vi "Set Parameter Properties.vi"(0 "custom device ref in":T1=18446744073709551615 format="%.0x", 1 "port sessions":T2 {"portConfiguration"."Rx_UDP"."Tx_UDP"."FilterMode" items=["FDX_RX_VL_FLT_DIS", "FDX_RX_VL_FLT_ENA ", "FDX_RX_VL_FLT_ENA_INV"]; "portConfiguration"."Rx_UDP"."Tx_UDP"."VLBufSize" format="%.0x"; "portConfiguration"."Rx_UDP"."Tx_UDP"."VerificationMode" items=["FDX_RX_VL_CHECK_ENA_DEFAULT"=65535, "FDX_RX_VL_CHECK_REDMAM"=16, "DX_RX_VL_CHECK_TRAFIC"=8, "FDX_RX_VL_CHECK_FRAMESIZE"=4, "FDX_RX_VL_CHECK_SNINTEG"=2, "FDX_RX_VL_CHECK_INVPAC"=1, "FDX_RX_VL_CHECK_DISA"=0]; "portConfiguration"."Tx_UDP"."tx_udp_setup"."interfaceID" format="%.0b"; "portConfiguration"."Tx_UDP"."tx_udp_setup"."NetSelect" items=["FDX_TX_FRAME_DLY_A"=0, "FDX_TX_FRAME_DLY_B"=1, "FDX_TX_FRAME_BOTH "=3, "FDX_TX_FRAME_ONLY_A"=4, "FDX_TX_FRAME_ONLY_B "=5]; "portConfiguration"."Rx_Monitor"."Strobe" items=["FDX_MON_STROBE_DIS", "FDX_MON_STROBE_STOP", "FDX_MON_STROBE_START"]; "portConfiguration"."Rx_Monitor"."CaptureMode" items=["FDX_MON_SINGLE ", "FDX_MON_CONTINUOUS", "FDX_MON_SELECTIVE", "FDX_MON_RECORDING", "FDX_MON_REROS", "FDX_MON_HMU"]; "portConfiguration"."Rx_Monitor"."DefaultCronoMode" items=["FDX_RX_DEFAULT_ENA_CNT", "FDX_RX_DEFAULT_MON_ENA_ALL", "FDX_RX_DEFAULT_MON_ENA_GOOD"]; "portConfiguration"."Tx_Generic"."Frame Headers"."Frame header"."PhysErrorInjection" items=["FDX_TX_FRAME_ERR_OFF", "FDX_TX_FRAME_ERR_CRC", "FDX_TX_FRAME_ERR_ALI", "FDX_TX_FRAME_ERR_PRE", "FDX_TX_FRAME_ERR_PHY"]; "portConfiguration"."Tx_Generic"."Frame Headers"."Frame header"."PayloadGenerationMode" items=["FDX_TX_FRAME_PGM_USER", "FDX_TX_FRAME_PGM_IP_PART", "FDX_TX_FRAME_PGM_IP_PART_TT", "FDX_TX_FRAME_PGM_IP_FULL", "FDX_TX_FRAME_PGM_IP_FULL_TT"]; "portConfiguration"."Tx_Generic"."Frame Headers"."Frame header"."PayloadBufferMode" items=["FDX_TX_FRAME_PBM_STD", "FDX_TX_FRAME_PBM_MAC", "FDX_TX_FRAME_PBM_UDP", "FDX_TX_FRAME_PBM_FULL"]; "portConfiguration"."Tx_Generic"."Frame Headers"."Frame header"."NetSelect" items=["FDX_TX_FRAME_DLY_A"=0, "FDX_TX_FRAME_DLY_B"=1, "FDX_TX_FRAME_BOTH "=3, "FDX_TX_FRAME_ONLY_A"=4, "FDX_TX_FRAME_ONLY_B "=5]; "portConfiguration"."Tx_Generic"."Frame Headers"."Frame header"."FrameStartMode" items=["FDX_TX_FRAME_START_IFG", "FDX_TX_FRAME_START_PGWT", "FDX_TX_FRAME_START_TRG", "FDX_TX_FRAME_START_TRG_D"]; "portConfiguration"."Tx_Generic"."tx_generic_setup"."StartMode" items=["FDX_STOP", "FDX_START", "FDX_START_TRG", "FDX_START_TIME"]; "boardSetup"."portConfig" items=["FDX_SINGLE", "FDX_REDUNDANT"]; "boardSetup"."portSpeed" items=["FDX_100MBIT", "FDX_10MBIT", "FDX_AUTO_100MBIT", "FDX_AUTO_10MBIT", "FDX_AUTO_ERROR", "FDX_1000MBIT"]}, 3 "error in":errorcluster) -> (7 "custom device ref out":T1=18446744073709551615 format="%.0x", 10 "error out":errorcluster)   [LabVIEW 2020, in "AIM ARINC 664 Scripting.lvlib"]
uses:
  AIM ARINC 664 Scripting.lvlib
  Import/_typedefs/Board Top Level Configuration.ctl
  Import/_typedefs/board_setup.ctl
  Import/_typedefs/port_configuration.ctl
  Import/_typedefs/port_setup.ctl
  Import/_typedefs/session_tx_generic.ctl
  Import/_typedefs/tx_generic_setup.ctl
  Import/_typedefs/frame_tx_generic.ctl
  Import/_typedefs/frame_tx_generic_seqNumberInit.ctl
  Import/_typedefs/frame_tx_generic_seqNumberOffset.ctl
  Import/_typedefs/frame_parameter.ctl
  Import/_typedefs/frame_parameter_definition.ctl
  Shared/Encoding (Arinc664).ctl
  Import/_typedefs/port_tx_udp_comm.ctl
  Import/_typedefs/port_tx_udp_sap.ctl
  Import/_typedefs/rx_udp_setup.ctl
  Import/_typedefs/port_rx_udp_comm.ctl
  Import/_typedefs/port_rx_udp_sap.ctl
  <vilib>/NI VeriStand/Custom Device API/Custom Device Item Ref.ctl
  Import/AIM ARINC 664 Import.lvlib
  <vilib>/NI VeriStand/Custom Device API/Custom Device API.lvlib
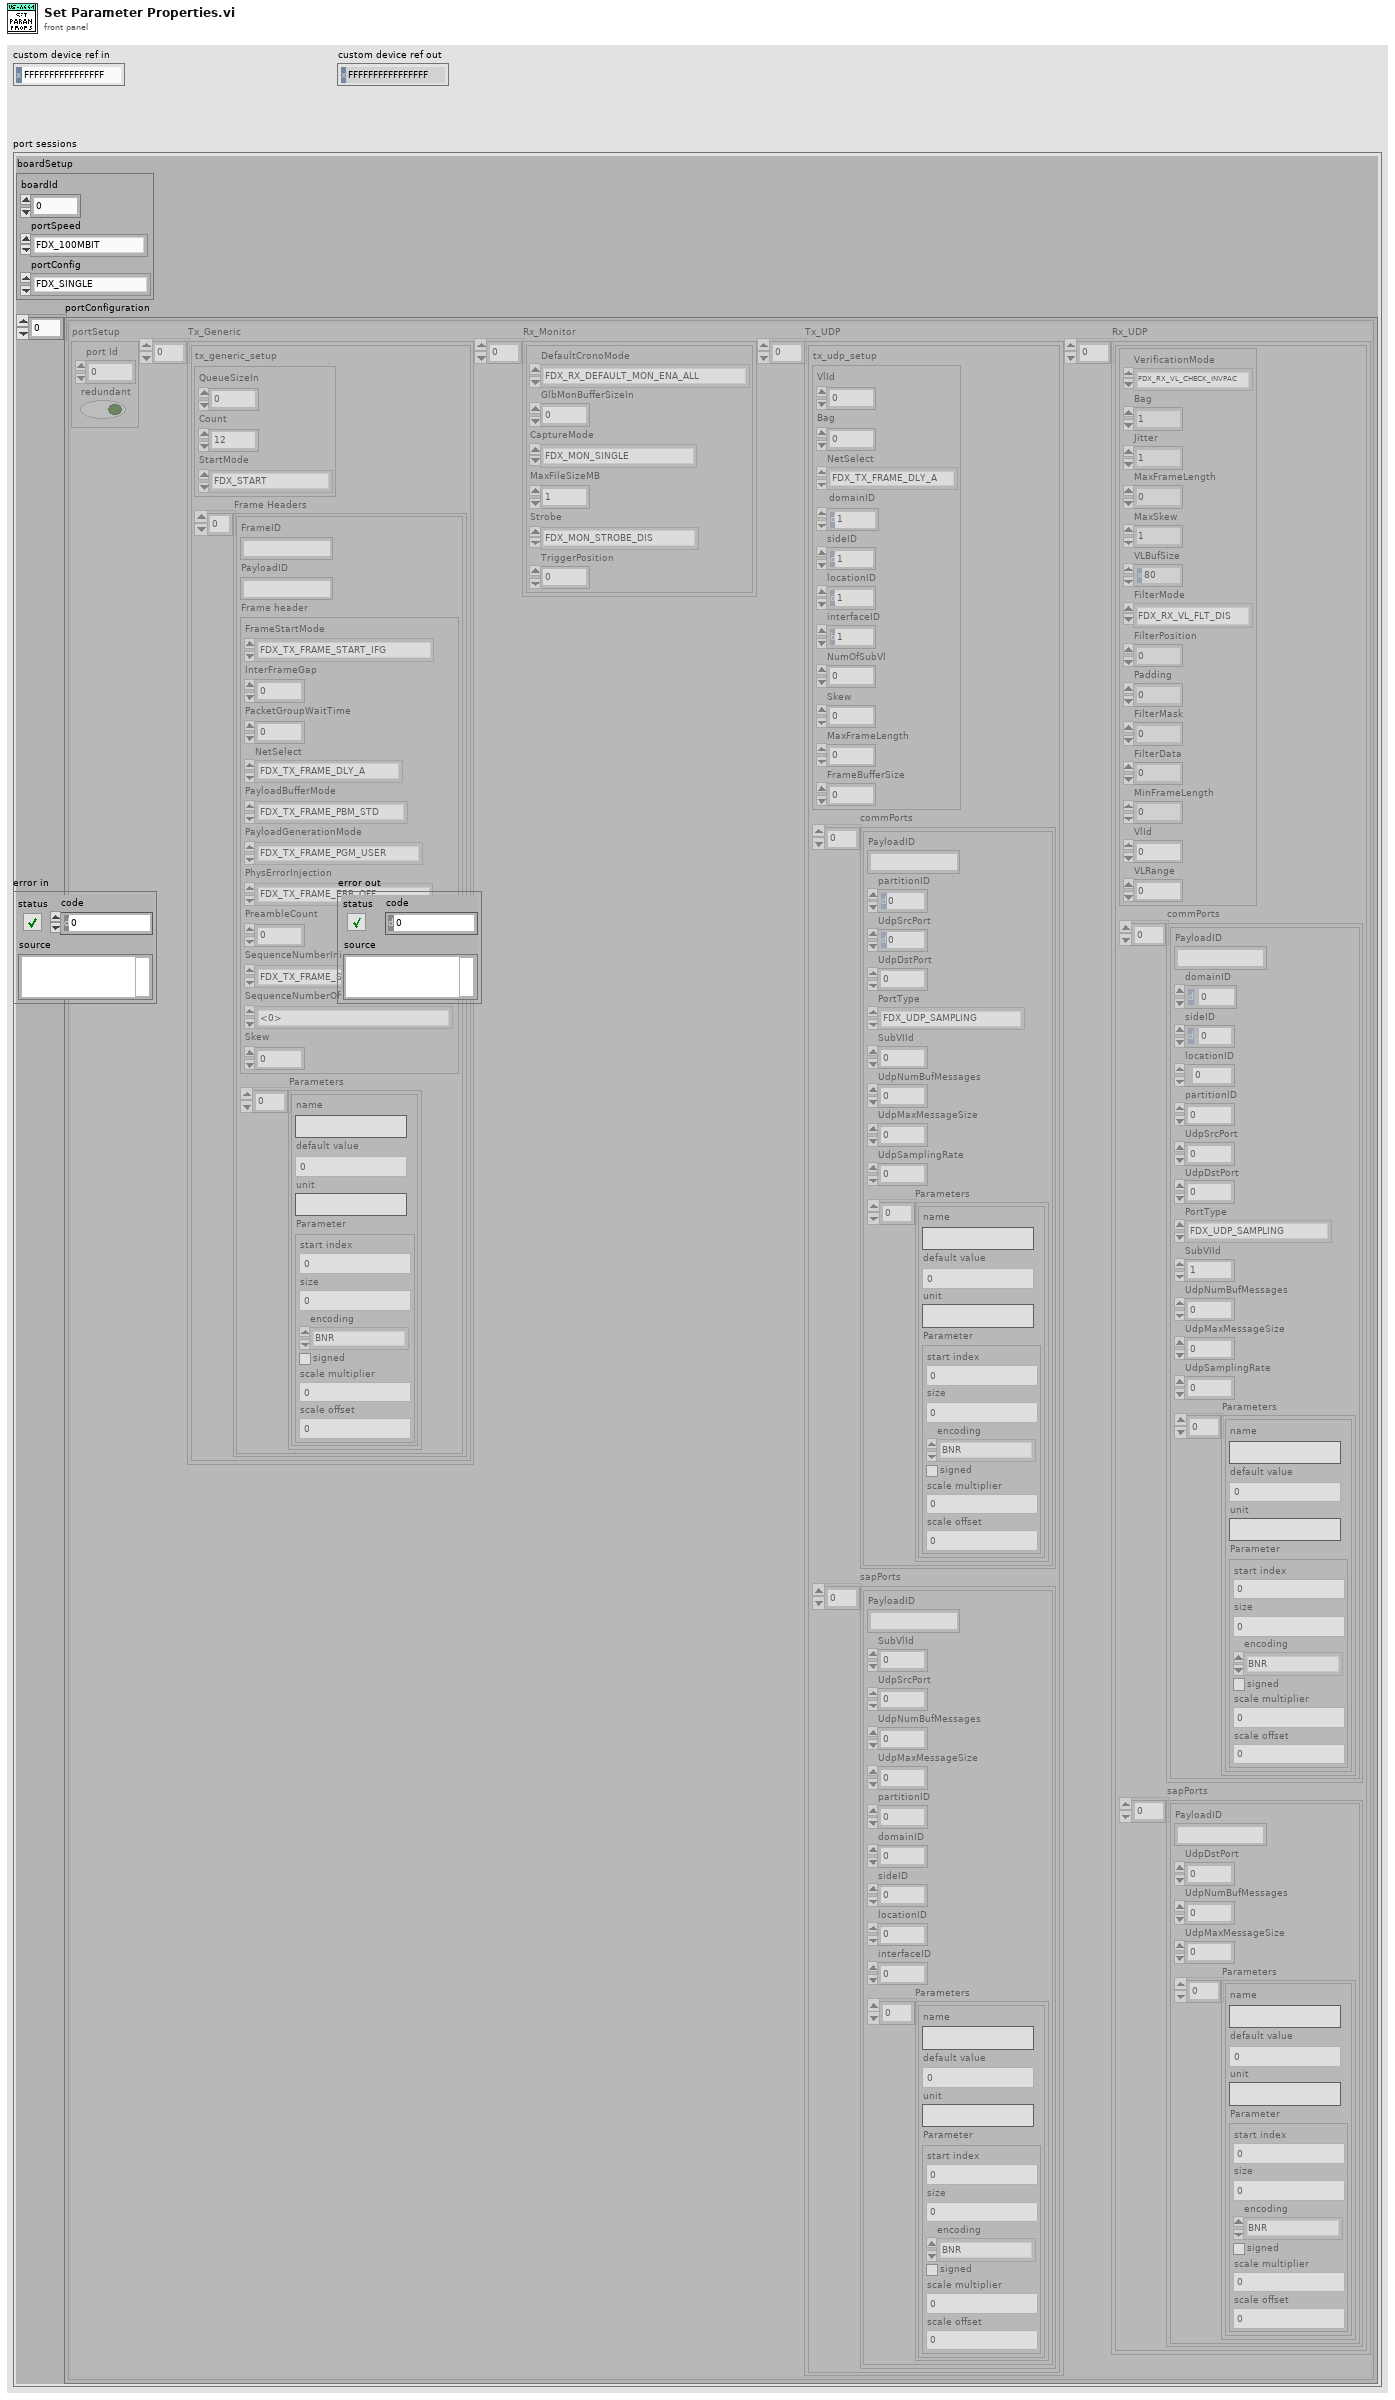
[diagram p1: front panel]
types:
  T1 = typedef "Custom Device API.lvlib/Custom Device Item Ref.ctl" = u64
  T2 = typedef "AIM ARINC 664 Import.lvlib/Board Top Level Configuration.ctl" = cluster{"boardSetup":T3, "portConfiguration":T4[]}
  T3 = typedef "AIM ARINC 664 Import.lvlib/board_setup.ctl" = cluster{"boardId":u32, "portSpeed":u32, "portConfig":u32}
  T4 = typedef "AIM ARINC 664 Import.lvlib/port_configuration.ctl" = cluster{"portSetup":T5, "Tx_Generic":T6[], "Rx_Monitor":cluster{"DefaultCronoMode":u32, "GlbMonBufferSizeIn":u32, "CaptureMode":u32, "MaxFileSizeMB":u32, "Strobe":u32, "TriggerPosition":u32}[], "Tx_UDP":cluster{"tx_udp_setup":cluster{"VlId":i32, "Bag":i32, "NetSelect":u32, "domainID":u8, "sideID":u8, "locationID":u8, "interfaceID":u8, "NumOfSubVl":u16, "Skew":u32, "MaxFrameLength":u32, "FrameBufferSize":u32}, "commPorts":T14[], "sapPorts":T15[]}[], "Rx_UDP":cluster{"Tx_UDP":T16, "commPorts":T17[], "sapPorts":T18[]}[]}
  T5 = typedef "AIM ARINC 664 Import.lvlib/port_setup.ctl" = cluster{"port Id":u32, "redundant":bool}
  T6 = typedef "AIM ARINC 664 Import.lvlib/session_tx_generic.ctl" = cluster{"tx_generic_setup":T7, "Frame Headers":T8[]}
  T7 = typedef "AIM ARINC 664 Import.lvlib/tx_generic_setup.ctl" = cluster{"QueueSizeIn":u32, "Count":i32, "StartMode":i32}
  T8 = typedef "AIM ARINC 664 Import.lvlib/frame_tx_generic.ctl" = cluster{"FrameID":string, "PayloadID":string, "Frame header":cluster{"FrameStartMode":i32, "InterFrameGap":i32, "PacketGroupWaitTime":i32, "NetSelect":u32, "PayloadBufferMode":i32, "PayloadGenerationMode":i32, "PhysErrorInjection":i32, "PreambleCount":i32, "SequenceNumberInit":T9, "SequenceNumberOffset":T10, "Skew":i32}, "Parameters":T11[]}
  T9 = typedef "AIM ARINC 664 Import.lvlib/frame_tx_generic_seqNumberInit.ctl" = i32
  T10 = typedef "AIM ARINC 664 Import.lvlib/frame_tx_generic_seqNumberOffset.ctl" = i32
  T11 = typedef "AIM ARINC 664 Import.lvlib/frame_parameter.ctl" = cluster{"name":string, "default value":dbl, "unit":string, "Parameter":T12}
  T12 = typedef "AIM ARINC 664 Import.lvlib/frame_parameter_definition.ctl" = cluster{"start index":i32, "size":i32, "encoding":T13, "signed":bool, "scale multiplier":dbl, "scale offset":dbl}
  T13 = typedef "Encoding (Arinc664).ctl" = u16
  T14 = typedef "AIM ARINC 664 Import.lvlib/port_tx_udp_comm.ctl" = cluster{"PayloadID":string, "partitionID":u8, "UdpSrcPort":u16, "UdpDstPort":u16, "PortType":enum16{"FDX_UDP_SAMPLING", "FDX_UDP_QUEUING"}, "SubVIId":u32, "UdpNumBufMessages":u32, "UdpMaxMessageSize":u32, "UdpSamplingRate":u32, "Parameters":T11[]}
  T15 = typedef "AIM ARINC 664 Import.lvlib/port_tx_udp_sap.ctl" = cluster{"PayloadID":string, "SubVlId":u8, "UdpSrcPort":u16, "UdpNumBufMessages":u32, "UdpMaxMessageSize":u32, "partitionID":u8, "domainID":u8, "sideID":u8, "locationID":u8, "interfaceID":u8, "Parameters":T11[]}
  T16 = typedef "AIM ARINC 664 Import.lvlib/rx_udp_setup.ctl" = cluster{"VerificationMode":u32, "Bag":u32, "Jitter":u32, "MaxFrameLength":u32, "MaxSkew":u32, "VLBufSize":u32, "FilterMode":u32, "FilterPosition":u32, "Padding":u32, "FilterMask":u32, "FilterData":u32, "MinFrameLength":u32, "VlId":u16, "VLRange":u32}
  T17 = typedef "AIM ARINC 664 Import.lvlib/port_rx_udp_comm.ctl" = cluster{"PayloadID":string, "domainID":u8, "sideID":u8, "locationID":u8, "partitionID":u8, "UdpSrcPort":u16, "UdpDstPort":u16, "PortType":enum16{"FDX_UDP_SAMPLING", "FDX_UDP_QUEUING"}, "SubVIId":u32, "UdpNumBufMessages":u32, "UdpMaxMessageSize":u32, "UdpSamplingRate":u32, "Parameters":T11[]}
  T18 = typedef "AIM ARINC 664 Import.lvlib/port_rx_udp_sap.ctl" = cluster{"PayloadID":string, "UdpDstPort":u16, "UdpNumBufMessages":u32, "UdpMaxMessageSize":u32, "Parameters":T11[]}
  T19 = cluster{"DefaultCronoMode":u32, "GlbMonBufferSizeIn":u32, "CaptureMode":u32, "MaxFileSizeMB":u32, "Strobe":u32, "TriggerPosition":u32}[]
  T20 = cluster{"tx_udp_setup":cluster{"VlId":i32, "Bag":i32, "NetSelect":u32, "domainID":u8, "sideID":u8, "locationID":u8, "interfaceID":u8, "NumOfSubVl":u16, "Skew":u32, "MaxFrameLength":u32, "FrameBufferSize":u32}, "commPorts":T14[], "sapPorts":T15[]}[]
  T21 = cluster{"Tx_UDP":T16, "commPorts":T17[], "sapPorts":T18[]}[]
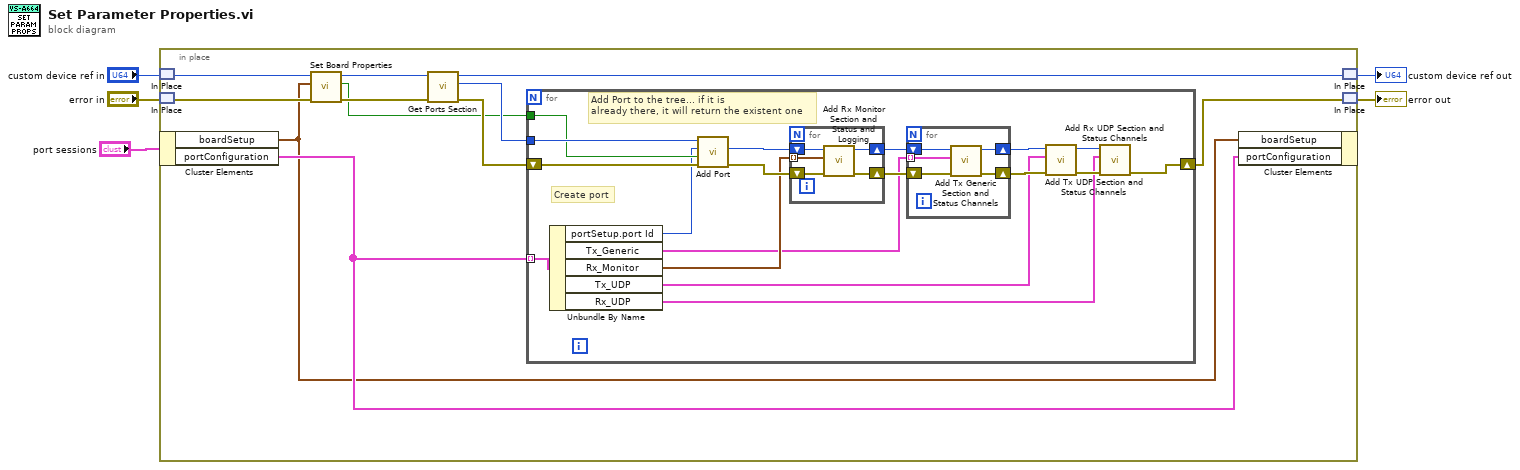
[diagram p0: block diagram]
diagram:
  n1 = in-place {
    n2 = in-place-match #1("custom device ref in") -> (w16:T1)
    n3 = in-place-match #2("error in") -> (w15:errorcluster)
    n4 = in-place-cluster #3("port sessions") -> ("boardSetup"=w6:T3, "portConfiguration"=w7:T4[])
    n5 = call "Set Board Properties.vi"("error in"=w15, "board setup"=w6, "custom device ref in"=w16) -> ("error out"=w11:errorcluster, "redundant?"=w10:bool, "custom device ref out"=w12:T1)  [unwired: 6 in]
    n6 = call "Get Ports Section.vi"("error in"=w11, "custom device ref"=w12) -> ("error out"=w13:errorcluster, "ports ref out"=w14:T1, "custom device ref out"=w9:T1)  [unwired: 6 in, 1 out]
    n7 = for {
      tunnel: w14 -> [w29]
      tunnel: w10 -> [w25]
      shift-right: [w30] -> w8
      shift-left: w13 -> [w27]
      tunnel: w7 -> [w28] mode=indexing
      # "Add Port to the tree... if it is \nalready there, it will return the existent one"
      # "Create port"
      n8 = Unbundle By Name(w28) -> ("portSetup.port Id"=w23:u32, "Tx_Generic"=w21:T6[], "Rx_Monitor"=w22:T19, "Tx_UDP"=w20:T20, "Rx_UDP"=w17:T21)
      n9 = call "Add Port.vi"("error in"=w27, "redundant ?"=w25, "port Id"=w23, "ports ref"=w29) -> ("error out"=w24:errorcluster, "port ref out"=w26:T1)  [unwired: 5 in, 1 out]
      n10 = for {
        tunnel: w22 -> [w40] mode=indexing
        shift-right: [w43] -> w33
        shift-left: w26 -> [w42]
        shift-right: [w44] -> w34
        shift-left: w24 -> [w41]
        n11 = call "Add Rx Monitor Section and Status and Logging.vi"("error in"=w41, "session_rx_monitor"=w40, "port ref"=w42) -> ("error out"=w44:errorcluster, "port ref out"=w43:T1)  [unwired: 7 in]
      }
      n12 = for {
        tunnel: w21 -> [w35] mode=indexing
        shift-right: [w37] -> w32
        shift-left: w34 -> [w39]
        shift-right: [w36] -> w31
        shift-left: w33 -> [w38]
        n13 = call "Add Tx Generic Section and Status Channels.vi"("error in"=w39, "Tx generic configuration"=w35, "port ref"=w38) -> ("error out"=w37:errorcluster, "port ref out"=w36:T1)  [unwired: 7 in]
      }
      n14 = call "Add Tx UDP Section and Status Channels.vi"("error in"=w32, "Tx UDP configuration"=w20, "port ref"=w31) -> ("error out"=w19:errorcluster, "port ref out"=w18:T1)  [unwired: 7 in]
      n15 = call "Add Rx UDP Section and Status Channels.vi"("error in"=w19, "Rx UDP configuration"=w17, "port ref"=w18) -> ("error out"=w30:errorcluster)  [unwired: 7 in, 1 out]
    }
    n16 = in-place-cluster #3("boardSetup"=w6, "portConfiguration"=w7) -> ()  [unwired: 1 out]
    n17 = in-place-match #1(w9) -> (→"custom device ref out":T1)
    n18 = in-place-match #2(w8) -> (→"error out":errorcluster)
  }
